vi "Top (FPGA)-1port.vi"() -> ()   [LabVIEW 2024]
uses:
  <vilib>/Platform/TimedLoop/XDataNode/wakeup.ctl
  <vilib>/Platform/TimedLoop/XDataNode/XDNodeRunTimeDep.lvlib
  <vilib>/Platform/TimedLoop/XDataNode/nitl_modes.ctl
  <vilib>/Platform/TimedLoop/XDataNode/timing_clust.ctl
  <vilib>/Platform/TimedLoop/XDataNode/XDataNode.xnode
  <instrlib>/_niInstr/FIFO Register Bus/v1/FPGA/niInstr FIFO Register Bus v1 FPGA.lvclass
  <instrlib>/_niInstr/Instruction Framework/v1/FPGA/Top Level Bus/Register Configuration/Register Configuration.lvclass
  <instrlib>/_niInstr/Instruction Framework/v1/FPGA/Collection Builder/Collection Builder.lvclass
  <instrlib>/_niInstr/Instruction Framework/v1/FPGA/Collection Builder/Parent Metadata.ctl
  <instrlib>/_niInstr/Instruction Framework/v1/FPGA/Collection Builder/niInstr Address Space Collection Builder v1 FPGA.lvlib
  PXIe-7903 Aurora Example.lvlib
  <vilib>/eio/EIONode/EIONode.xnode
  Utilities/FPGA/Aurora64b66b Utilities FPGA.lvlib
  <instrlib>/_niInstr/Basic Elements/v1/FPGA/niInstr Basic Elements v1 FPGA.lvlib
  <vilib>/rvi/eio/common/nirviEmuTemplateMethod_errors.vi
  <instrlib>/_niInstr/Aurora64b66b/v1/FPGA/Buffered/Aurora64b66b Buffered.lvclass
panel:
  in  "port 0 enable":bool
  out "port 0 mismatch count":u64
  in  "port 0 rx throttle":u16
  in  "tb reset":bool
  out "flexrio.module.io error 0":i32
  out "flexrio.module.io ready 0":bool
  in  "fifo reg bus ctrl 0":u32
  out "fifo reg bus status 0":u32
  out "fifo reg bus data 0":u64
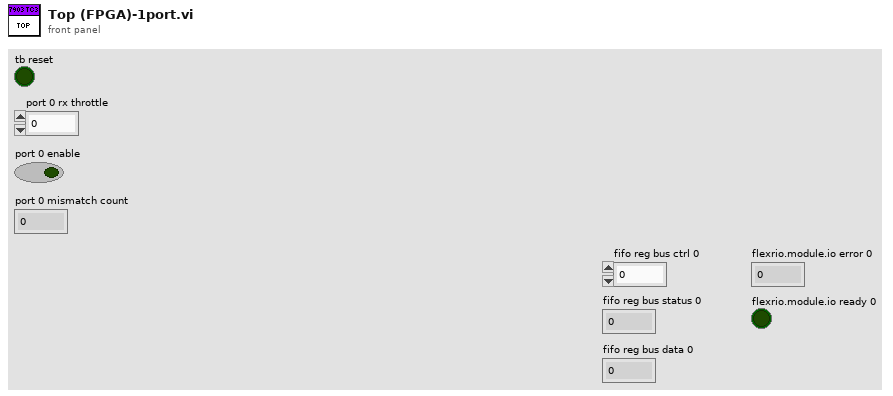
[diagram p1: front panel]
types:
  T1 = typedef "niInstr Address Space Collection Builder v1 FPGA.lvlib/Parent Metadata.ctl" = cluster{"UID":u16, "version":u16, "oldest compatible version":u16}
  T2 = typedef "XDNodeRunTimeDep.lvlib/timing_clust.ctl" = cluster{"Expected End [f-1]":u64, "Actual End [f-1]":u64, "Finished Late? [f-1]":bool, "Expected End [i-1]":u64, "Actual End [i-1]":u64, "Finished Late? [i-1]":bool, "Expected Start [i]":u64, "Actual Start [i]":u64, "Expected Start [f]":u64, "Actual Start [f]":u64, "Source Name":string, "Structure Name":string, "Period":i64, "Deadline":i64, "Offset":i64, "Start":i64, "Priority":i32, "Timeout":i32, "Mode":T3, "Wakeup Reason":T4, "Error":errorcluster, "Source Type":string, "Secondary Source Type":string, "Global End Time":u64, "Global Start Time":u64, "Frame Duration":u64, "Iteration Duration":u64, "Assigned CPU":i32, "I/O Scan Engine Mode":u32}
  T3 = typedef "XDNodeRunTimeDep.lvlib/nitl_modes.ctl" = enum32{"No Change", "Process missed periods, maintain original phase", "Discard missed periods, maintain original phase", "Process missed periods, ignore original phase", "Discard missed periods, ignore original phase"}
  T4 = typedef "XDNodeRunTimeDep.lvlib/wakeup.ctl" = enum32{"Normal", "Aborted", "Asynchronous wakeup", "Timing source error", "Timed loop error", "Timeout"}
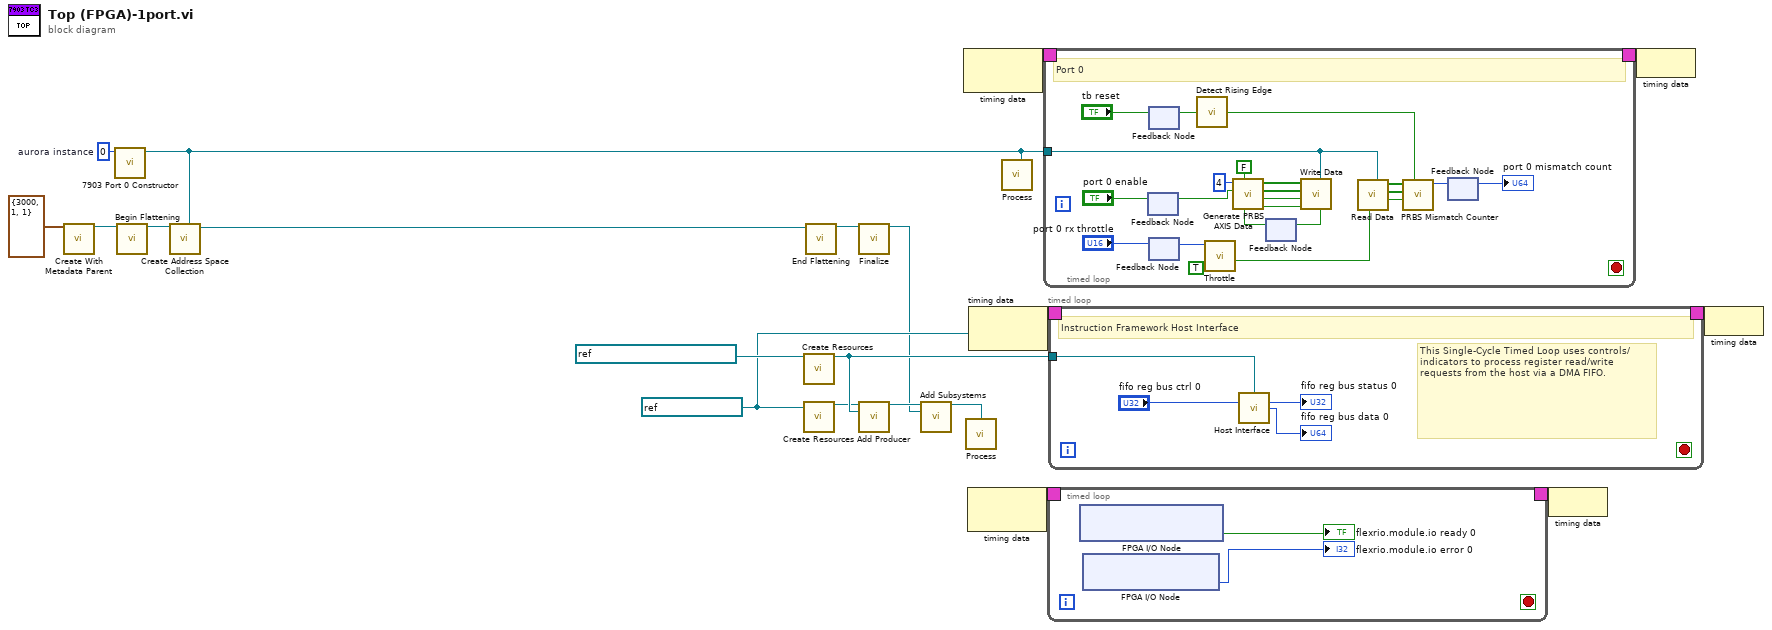
[diagram p0: block diagram]
diagram:
  w5 = u8 0  # aurora instance
  w15 = refnum<k21> "80 MHz Clock" ("Source Name")
  n1 = call <instrlib>:"Create With Metadata Parent.vi"("parent metadata"=T1 {"UID"=3000, "version"=1, "oldest compatible version"=1}) -> ("collection builder"=w14:refnum<class "Collection Builder.lvclass">)  [unwired: 14 in]
  n2 = call "7903 Port 0 Constructor.vi"("aurora instance (0)"=w5) -> ("aurora64b66b buffered"=w2:refnum<class "Aurora64b66b Buffered.lvclass">)  [unwired: 10 in]
  n3 = call <instrlib>:"Begin Flattening.vi"("collection builder in"=w14) -> ("collection builder out"=w8:refnum<class "Collection Builder.lvclass">)  [unwired: 14 in]
  n4 = call-dynamic "Create Address Space Collection.vi"("aurora64b66b basic"=w2, "collection builder in"=w8) -> ("collection builder out"=w1:refnum<class "Collection Builder.lvclass">)  [unwired: 9 in]
  n5 = call <instrlib>:"Create Resources.vi"("instruction fifo"=refnum<k21> "reg.host instruction fifo 0" ("FIFO")) -> ("fifo register bus"=w17:refnum<class "niInstr FIFO Register Bus v1 FPGA.lvclass">)  [unwired: 14 in]
  n6 = call <instrlib>:"Create Resources.vi"("register clock"=w15) -> ("register configuration"=w16:refnum<class "Register Configuration.lvclass">)  [unwired: 14 in]
  n7 = call <instrlib>:"End Flattening.vi"("collection builder in"=w1) -> ("collection builder out"=w13:refnum<class "Collection Builder.lvclass">)  [unwired: 14 in]
  n8 = call <instrlib>:"Finalize.vi"("collection builder in"=w13) -> ("address space collection"=w9:refnum<class "Address Space Collection.lvclass">)  [unwired: 14 in]
  n9 = call-dynamic "Add Producer.vi"("register configuration in"=w16, "instruction producer"=w17) -> ("register configuration out"=w11:refnum<class "Register Configuration.lvclass">)  [unwired: 13 in]
  n10 = call-dynamic "Add Subsystems.vi"("register configuration in"=w11, "subsystems"=w9) -> ("register configuration out"=w10:refnum<class "Register Configuration.lvclass">)  [unwired: 13 in]
  n11 = node-c288() -> (w4:T2)  [unwired: 1 in]
  n12 = call-dynamic "Process.vi"("register configuration"=w10) -> ()  [unwired: 15 in]
  n13 = node-c288() -> (w7:T2)  [unwired: 1 in]
  n14 = node-c288(w15) -> (w20:T2)
  n15 = call-dynamic "Process.vi"("aurora64b66b buffered"=w2) -> ()  [unwired: 11 in]
  n16 = timed-loop {
    timing: w4 -> [_]
    timing-out: [_] -> w3
    tunnel: w2 -> [w25]
    stop <- _ stop-if-true
    # "Port 0"
    n17 = feedback #1() -> (w21:bool)  [unwired: 1 in]
    n18 = feedback-in #1("port 0 enable") -> ()
    n19 = feedback-in #2("tb reset") -> ()
    n20 = feedback #2() -> (w26:bool)  [unwired: 1 in]
    n21 = feedback #3() -> (w29:u16)  [unwired: 1 in]
    n22 = feedback-in #3("port 0 rx throttle") -> ()
    n23 = call <instrlib>:"Detect Rising Edge.vi"("signal"=w26) -> ("edge detected"=w41:bool)  [unwired: 14 in]
    n24 = call "Throttle.vi"("request data"=TRUE ("Request Data"), "throttle"=w29) -> ("throttled request"=w34:bool)  [unwired: 9 in]
    n25 = feedback #4() -> (w39:bool)  [unwired: 1 in]
    n26 = call "Generate PRBS AXIS Data.vi"("ready for output"=w39, "reset"=FALSE, "enable"=w21, "number of lanes"=u8 4) -> ("tlast"=w35:bool, "tvalid"=w36:bool, "tkeep"=w37:bool[], "tdata"=w38:bool[])  [unwired: 4 in]
    n27 = call-dynamic "Write Data.vi"("aurora64b66b buffered"=w25, "tlast"=w35, "input valid"=w36, "tkeep"=w37, "tdata"=w38) -> ("ready for input"=w40:bool)  [unwired: 6 in]
    n28 = feedback-in #4(w40) -> ()
    n29 = call-dynamic "Read Data.vi"("aurora64b66b buffered"=w25, "ready for output"=w34) -> ("output valid"=w31:bool, "tkeep"=w32:bool[], "tdata"=w33:bool[])  [unwired: 6 in, 1 out]
    n30 = call "PRBS Mismatch Counter.vi"("reset mismatch count"=w41, "input valid"=w31, "tkeep"=w32, "data in"=w33) -> ("mismatch count"=w42:u64)  [unwired: 7 in]
    n31 = feedback-in #5(w42) -> ()
    n32 = feedback #5() -> (→"port 0 mismatch count":u64)  [unwired: 1 in]
  }
  n33 = timed-loop {
    timing: w7 -> [_]
    timing-out: [_] -> w6
    stop <- _ stop-if-true
    n34 = xnode "FPGA I/O Node"() -> ("IO Socket.IO Ready"=→"flexrio.module.io ready 0":bool)  [unwired: 1 in, 1 out]
    n35 = xnode "FPGA I/O Node"() -> ("IO Socket.IO Error"=→"flexrio.module.io error 0":i32)  [unwired: 1 in, 1 out]
  }
  n36 = timed-loop {
    timing: w20 -> [_]
    timing-out: [_] -> w19
    tunnel: w17 -> [w50]
    stop <- _ stop-if-true
    # "This Single-Cycle Timed Loop uses controls/indicators to process register read/write requests from the host via a DMA FIFO."
    # "Instruction Framework Host Interface"
    n37 = call <instrlib>:"Host Interface.vi"("fifo register bus"=w50, "fifo reg bus ctrl 0"="fifo reg bus ctrl 0") -> ("fifo reg bus status 0"=→"fifo reg bus status 0":u32, "fifo reg bus data 0"=→"fifo reg bus data 0":u64)  [unwired: 12 in]
  }
  n38 = node-c288(w6) -> ()
  n39 = node-c288(w3) -> ()
  n40 = node-c288(w19) -> ()
